vi "SamplePythonGenerators.vi"() -> ()   [LabVIEW 2016]
uses:
  VIs/uPythonX/PythonData.ctl
  VIs/uPythonX/uPythonX.xctl
  VIs/Console/ConsoleXControl.xctl
panel:
  in  "stop":bool
  out "Console":string(xcontrol)
  out "uPythonX":T1(xcontrol)
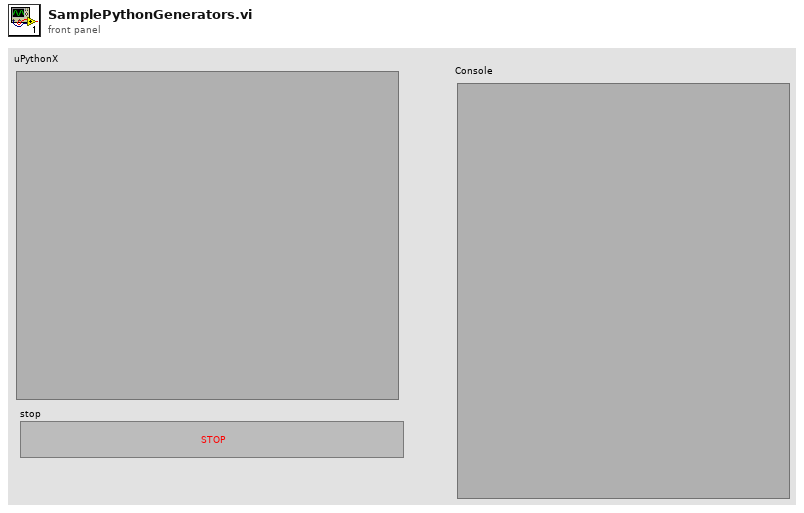
[diagram p1: front panel]
types:
  T1 = cluster{"VISA Refnum in":refnum<visa-resource-name>, "Python Code":string}
  T2 = typedef "uPythonX.xctl/PythonData.ctl" = cluster{"Port":refnum<visa-resource-name>, "All Code":string}
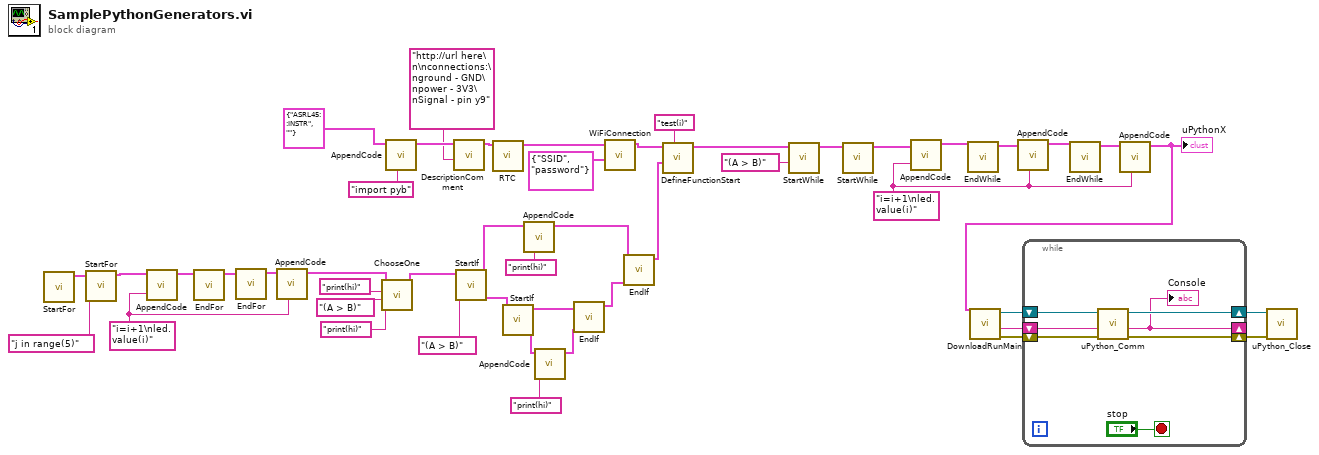
[diagram p0: block diagram]
diagram:
  w30 = "i=i+1\nled.value(i)" ("New Code")
  w39 = "i=i+1\nled.value(i)" ("New Code")
  n1 = call "StartFor.vi"() -> ("Data Out"=w36:T2)  [unwired: 11 in]
  n2 = call "StartFor.vi"("Comparison"="j in range(5)", "Data In"=w36) -> ("Data Out"=w33:T2)  [unwired: 9 in]
  n3 = call "AppendCode.vi"("New Code"=w30, "Data In"=w33) -> ("Data Out"=w34:T2)  [unwired: 9 in]
  n4 = call "EndFor.vi"("Data In"=w34) -> ("Data Out"=w35:T2)  [unwired: 10 in]
  n5 = call "EndFor.vi"("Data In"=w35) -> ("Data Out"=w31:T2)  [unwired: 10 in]
  n6 = call "AppendCode.vi"("New Code"=w30, "Data In"=w31) -> ("Data Out"=w5:T2)  [unwired: 9 in]
  n7 = call "ChooseOne.vi"("False Code"="print(hi)" ("New Code"), "Comparison"="(A > B)", "True Code"="print(hi)" ("New Code"), "Data In"=w5) -> ("Data Out"=w9:T2)  [unwired: 7 in]
  n8 = call "AppendCode.vi"("New Code"="import pyb", "Data In"=T2 {"Port"="ASRL45::INSTR", "All Code"=""}) -> ("Data Out"=w4:T2)  [unwired: 9 in]
  n9 = call "DescriptionComment.vi"("Description"="http://url here\n\nconnections:\nground - GND\npower - 3V3\nSignal - pin y9", "Data In"=w4) -> ("Data Out"=w2:T2)  [unwired: 9 in]
  n10 = call "StartIf.vi"("Comparison"="(A > B)", "Data In"=w9) -> ("False Out"=w23:T2, "True Out"=w28:T2)  [unwired: 8 in]
  n11 = call "RTC.vi"("Data In"=w2) -> ("Data Out"=w1:T2)  [unwired: 10 in]
  n12 = call "StartIf.vi"("Data In"=w23) -> ("False Out"=w21:T2, "True Out"=w19:T2)  [unwired: 9 in]
  n13 = call "AppendCode.vi"("New Code"="print(hi)", "Data In"=w28) -> ("Data Out"=w25:T2)  [unwired: 9 in]
  n14 = call "AppendCode.vi"("New Code"="print(hi)", "Data In"=w21) -> ("Data Out"=w20:T2)  [unwired: 9 in]
  n15 = call "EndIf.vi"("False In"=w20, "True In"=w19) -> ("Data Out"=w22:T2)  [unwired: 9 in]
  n16 = call "WiFiConnection.vi"("Login"=cluster{"SSID":string, "password":string} {"SSID"="SSID", "password"="password"}, "Data In"=w1) -> ("Data Out"=w18:T2)  [unwired: 9 in]
  n17 = call "EndIf.vi"("False In"=w22, "True In"=w25) -> ("Data Out"=w24:T2)  [unwired: 9 in]
  n18 = call "DefineFunctionStart.vi"("Function name"="test(i)", "Function"=w24, "Data In"=w18) -> ("Data Out"=w38:T2)  [unwired: 8 in]
  n19 = call "StartWhile.vi"("Comparison"="(A > B)", "Data In"=w38) -> ("Data Out"=w43:T2)  [unwired: 9 in]
  n20 = call "StartWhile.vi"("Data In"=w43) -> ("Data Out"=w42:T2)  [unwired: 10 in]
  n21 = call "AppendCode.vi"("New Code"=w39, "Data In"=w42) -> ("Data Out"=w44:T2)  [unwired: 9 in]
  n22 = call "EndWhile.vi"("Data In"=w44) -> ("Data Out"=w41:T2)  [unwired: 10 in]
  n23 = call "AppendCode.vi"("New Code"=w39, "Data In"=w41) -> ("Data Out"=w40:T2)  [unwired: 9 in]
  n24 = call "EndWhile.vi"("Data In"=w40) -> ("Data Out"=w45:T2)  [unwired: 10 in]
  n25 = call "AppendCode.vi"("New Code"=w39, "Data In"=w45) -> ("Data Out"=w11:T2)  [unwired: 9 in]
  "uPythonX" <- w11
  n26 = call "DownloadRunMain.vi"("Data In"=w11) -> ("error out"=w12:errorcluster, "Reply"=w13:string, "VISA Refnum out"=w14:refnum<visa-resource-name>)  [unwired: 8 in]
  n27 = while {
    shift-right: [w51] -> w15
    shift-left: w12 -> [w54]
    shift-right: [w50] -> w16
    shift-left: w14 -> [w52]
    shift-right: [w48] -> _
    shift-left: w13 -> [w53]
    stop <- "stop" stop-if-true
    n28 = call "uPython_Comm.vi"("error in (no error)"=w54, "Console In"=w53, "VISA Refnum in"=w52) -> ("error out"=w51:errorcluster, "Console Out"=w48:string, "VISA out"=w50:refnum<visa-resource-name>)  [unwired: 4 in, 2 out]
    "Console" <- w48
  }
  n29 = call "uPython_Close.vi"("error in"=w15, "VISA  in"=w16) -> ()  [unwired: 8 in, 2 out]
